vi "DRC Send Command.vi"(3 "error in (no error)":errorcluster, 4 "Input":dbl min=0.0 format="%.3f", 5 "StringInput":string, 6 "Command":T1(ring)) -> (0 "error out":errorcluster, 1 "Output":dbl format="%.2f", 2 "Response":string)   [LabVIEW 2019]
uses:
  GL_DRC_GPIBadd.vi
  GL_DRCtype.vi
  GL_DRCchannel.vi
panel:
  out "CHANNEL":bool
  out "CONTROLLER TYPE":bool
  out "GPIB Address":string
  # "setpoint, heater value"
  # "temperature,etc."
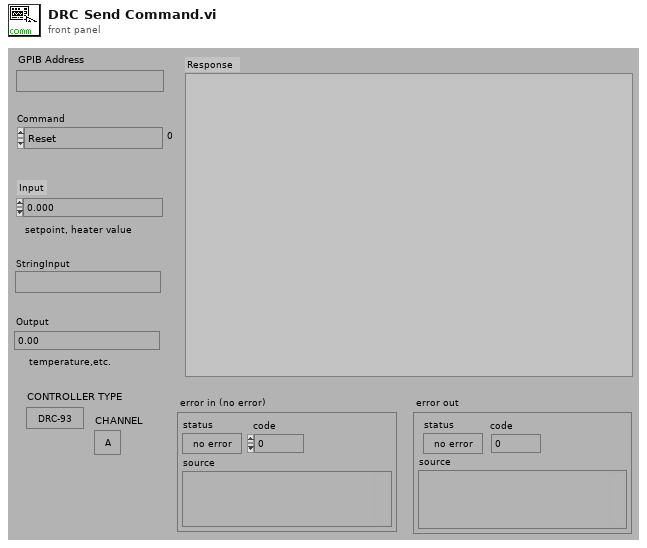
[diagram p1: front panel]
types:
  T1 = enum16{"Reset", "Raw_WriteRead", "ReadTemp", "WriteSetPoint", "ReadSetPoint", "ManualHeatPwr", "HeaterOff", "SetHeaterScale", "SetProportional(gain)", "SetIntegrate(reset)", "SetDerivative(rate)", "SendCalibration", "ReadCalibration", "SelectCurve", "GetControlInfo", "Change units", "GetDCSP_Reading", "GetPIDR_Reading", "ZeroNonVol_Mem"}
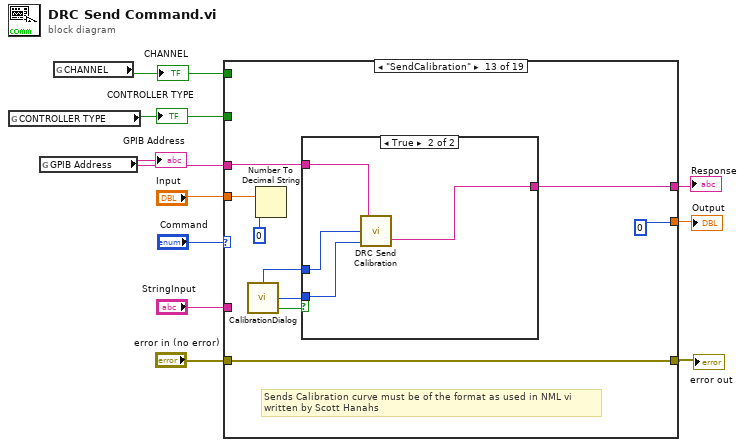
[diagram p0: block diagram]
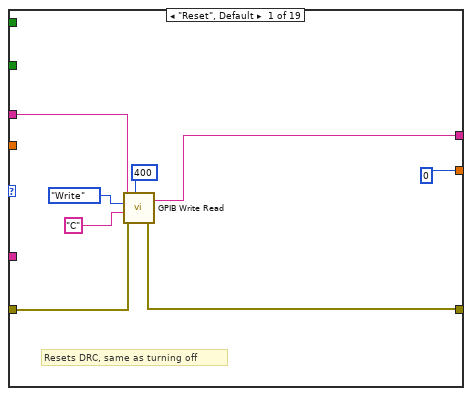
[diagram p2: hidden frame]
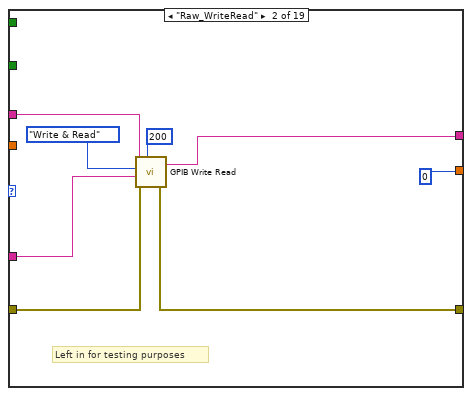
[diagram p3: hidden frame]
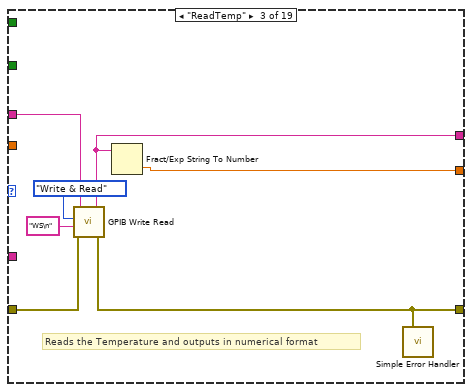
[diagram p4: hidden frame]
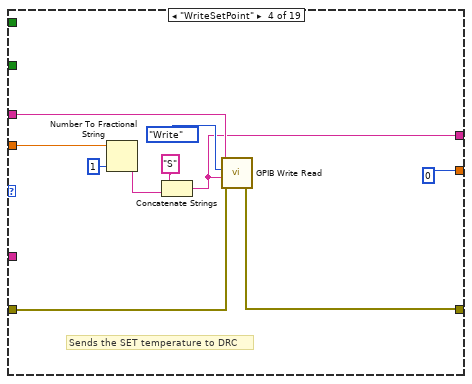
[diagram p5: hidden frame]
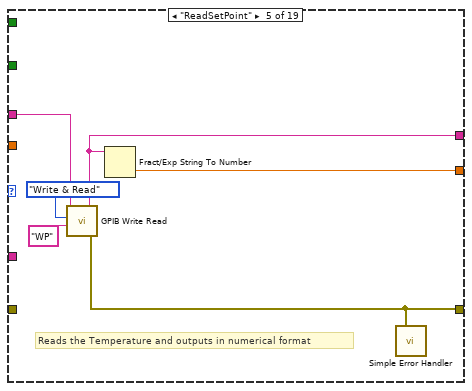
[diagram p6: hidden frame]
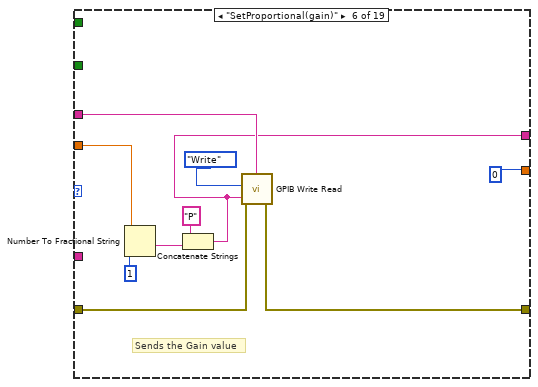
[diagram p7: hidden frame]
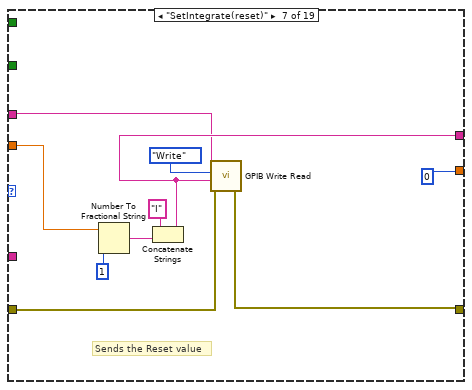
[diagram p8: hidden frame]
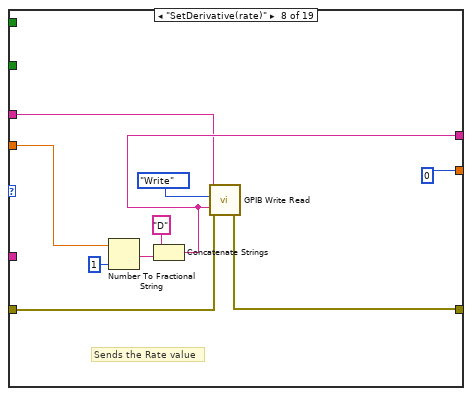
[diagram p9: hidden frame]
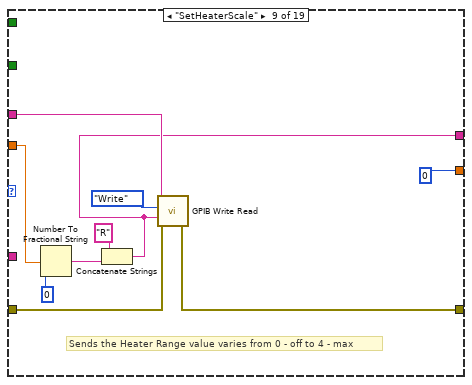
[diagram p10: hidden frame]
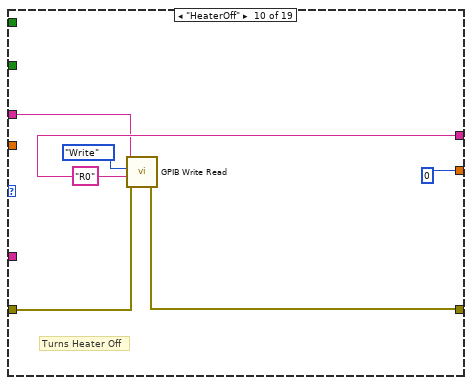
[diagram p11: hidden frame]
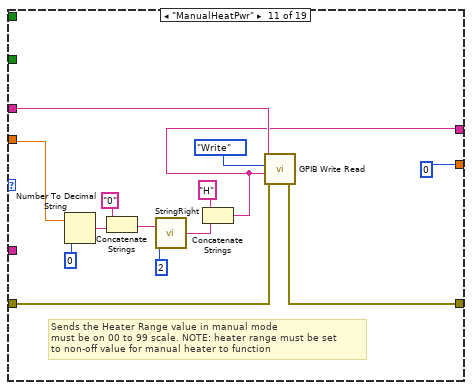
[diagram p12: hidden frame]
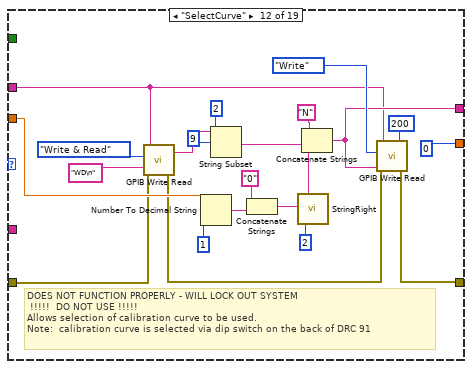
[diagram p13: hidden frame]
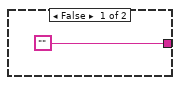
[diagram p14: hidden frame]
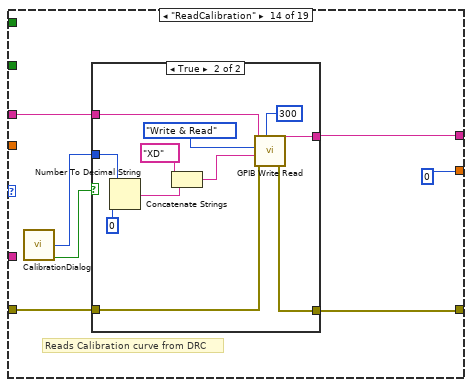
[diagram p15: hidden frame]
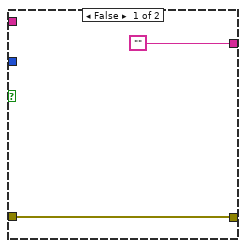
[diagram p16: hidden frame]
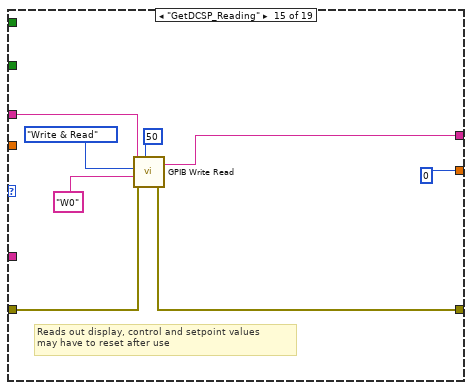
[diagram p17: hidden frame]
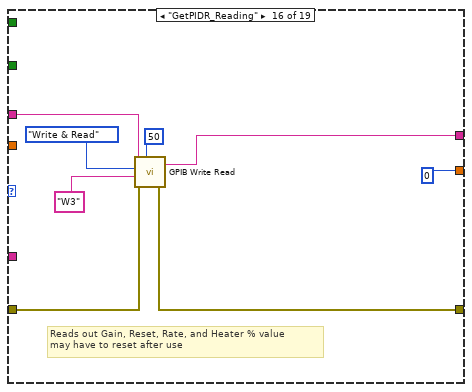
[diagram p18: hidden frame]
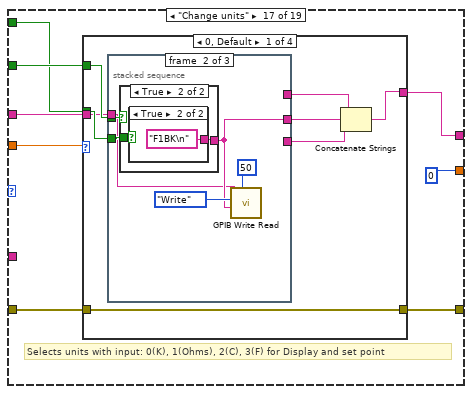
[diagram p19: hidden frame]
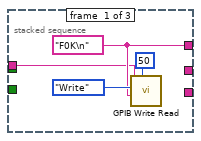
[diagram p20: hidden frame]
diagram:
  n1 = global read "GL_DRCtype.vi" "CONTROLLER TYPE"() -> (w2:bool)
  "CONTROLLER TYPE" <- w2
  n2 = global read "GL_DRC_GPIBadd.vi" "GPIB Address"() -> (w3:string)
  "GPIB Address" <- w3
  n3 = global read "GL_DRCchannel.vi" "CHANNEL"() -> (w1:bool)
  "CHANNEL" <- w1
  n4 = case shown="\"SendCalibration\"" "Command" {
    tunnel: [w15 w21 w30 w34 w46 w52 w64 w74 w82 w94 w98 w117 w137 w150 w168 w175 w184 w329 "Non-Volatile memory has been reinitialized"] -> w10
    tunnel: "StringInput" -> [_ w20 _ _ _ _ _ _ _ _ _ _ _ _ _ _ _ _ _]
    tunnel: "Input" -> [_ _ _ w38 _ w56 w66 w76 w86 _ w107 w122 w138 _ _ _ w189 _ _]
    tunnel: "error in (no error)" -> [w17 w23 w33 w37 _ w53 w62 w72 w83 w92 w99 w119 w136 w151 w170 w177 w188 w333 w340]
    tunnel: w2 -> [_ _ _ _ _ _ _ _ _ _ _ _ _ _ _ _ w187 w327 _]
    tunnel: w1 -> [_ _ _ _ _ _ _ _ _ _ _ _ _ _ _ _ w186 _ _]
    tunnel: [w12 w22 w27 w36 w44 w51 w61 w71 w81 w91 w97 w111 w136 w149 w169 w178 w185 w330 w338] -> w5
    tunnel: w3 -> [w18 w24 w31 w39 w49 w54 w63 w73 w84 w93 w100 w116 w140 w152 w171 w176 w183 w332 w341]
    tunnel: [0 0 w28 0 w45 0 0 0 0 0 0 0 0 0 0 0 0 0 0] -> w4
    frame "Reset", Default {
      # "Resets DRC, same as turning off"
      n5 = call "GPIB Write Read.vi"("GPIB address"=w18, "Action"=enum16{"Write", "Read", "Write & Read"}."Write" ("y"), "String to Write"="C" ("InputString"), "error in (no error)"=w17, "wait (mS)"=400) -> ("String Read"=w15:string, "error out"=w12:errorcluster)
    }
    frame "Raw_WriteRead" {
      # "Left in for testing purposes"
      n6 = call "GPIB Write Read.vi"("GPIB address"=w24, "Action"=enum16{"Write", "Read", "Write & Read"}."Write & Read", "String to Write"=w20, "error in (no error)"=w23, "wait (mS)"=200) -> ("String Read"=w21:string, "error out"=w22:errorcluster)
    }
    frame "ReadTemp" {
      # "Reads the Temperature and outputs in numerical format"
      n7 = call "GPIB Write Read.vi"("GPIB address"=w31, "Action"=enum16{"Write", "Read", "Write & Read"}."Write & Read", "String to Write"="WS\n", "error in (no error)"=w33) -> ("String Read"=w30:string, "error out"=w27:errorcluster)  [unwired: 1 in]
      n8 = Fract/Exp String To Number(string=w30) -> (number=w28:dbl)  [unwired: 3 in, 1 out]
      n9 = call <vilib>:"Simple Error Handler.vi"("error in (no error)"=w27) -> ()  [unwired: 4 in, 5 out]
    }
    frame "WriteSetPoint" {
      # "Sends the SET temperature to DRC"
      n10 = Number To Fractional String(number=w38, precision (6)=i16 1) -> (F-format string=w42:string)  [unwired: 2 in]
      n11 = Concatenate Strings("S", w42) -> (w34:string)
      n12 = call "GPIB Write Read.vi"("GPIB address"=w39, "Action"=enum16{"Write", "Read", "Write & Read"}."Write" ("y"), "String to Write"=w34, "error in (no error)"=w37) -> ("error out"=w36:errorcluster)  [unwired: 1 in, 1 out]
    }
    frame "ReadSetPoint" {
      # "Reads the Temperature and outputs in numerical format"
      n13 = call "GPIB Write Read.vi"("GPIB address"=w49, "Action"=enum16{"Write", "Read", "Write & Read"}."Write & Read", "String to Write"="WP") -> ("String Read"=w46:string, "error out"=w44:errorcluster)  [unwired: 2 in]
      n14 = Fract/Exp String To Number(string=w46) -> (number=w45:dbl)  [unwired: 3 in, 1 out]
      n15 = call <vilib>:"Simple Error Handler.vi"("error in (no error)"=w44) -> ()  [unwired: 4 in, 5 out]
    }
    frame "SetProportional(gain)" {
      # "Sends the Gain value"
      n16 = Number To Fractional String(number=w56, precision (6)=i16 1) -> (F-format string=w58:string)  [unwired: 2 in]
      n17 = Concatenate Strings("P", w58) -> (w52:string)
      n18 = call "GPIB Write Read.vi"("GPIB address"=w54, "Action"=enum16{"Write", "Read", "Write & Read"}."Write" ("y"), "String to Write"=w52, "error in (no error)"=w53) -> ("error out"=w51:errorcluster)  [unwired: 1 in, 1 out]
    }
    frame "SetIntegrate(reset)" {
      # "Sends the Reset value"
      n19 = Number To Fractional String(number=w66, precision (6)=i16 1) -> (F-format string=w68:string)  [unwired: 2 in]
      n20 = Concatenate Strings("I", w68) -> (w64:string)
      n21 = call "GPIB Write Read.vi"("GPIB address"=w63, "Action"=enum16{"Write", "Read", "Write & Read"}."Write" ("y"), "String to Write"=w64, "error in (no error)"=w62) -> ("error out"=w61:errorcluster)  [unwired: 1 in, 1 out]
    }
    frame "SetDerivative(rate)" {
      # "Sends the Rate value"
      n22 = Number To Fractional String(number=w76, precision (6)=i16 1) -> (F-format string=w78:string)  [unwired: 2 in]
      n23 = Concatenate Strings("D", w78) -> (w74:string)
      n24 = call "GPIB Write Read.vi"("GPIB address"=w73, "Action"=enum16{"Write", "Read", "Write & Read"}."Write" ("y"), "String to Write"=w74, "error in (no error)"=w72) -> ("error out"=w71:errorcluster)  [unwired: 1 in, 1 out]
    }
    frame "SetHeaterScale" {
      # "Sends the Heater Range value varies from 0 - off to 4 - max"
      n25 = Number To Fractional String(number=w86, precision (6)=i16 0) -> (F-format string=w88:string)  [unwired: 2 in]
      n26 = Concatenate Strings("R", w88) -> (w82:string)
      n27 = call "GPIB Write Read.vi"("GPIB address"=w84, "Action"=enum16{"Write", "Read", "Write & Read"}."Write" ("y"), "String to Write"=w82, "error in (no error)"=w83) -> ("error out"=w81:errorcluster)  [unwired: 1 in, 1 out]
    }
    frame "HeaterOff" {
      w94 = "R0"
      # "Turns Heater Off"
      n28 = call "GPIB Write Read.vi"("GPIB address"=w93, "Action"=enum16{"Write", "Read", "Write & Read"}."Write" ("y"), "String to Write"=w94, "error in (no error)"=w92) -> ("error out"=w91:errorcluster)  [unwired: 1 in, 1 out]
    }
    frame "ManualHeatPwr" {
      # "Sends the Heater Range value in manual mode \nmust be on 00 to 99 scale. NOTE: heater range must be set \nto non-off value for manual heater to function"
      n29 = Number To Decimal String(number=w107, width (-)=i16 0 ("precision (6)")) -> (decimal integer string=w103:string)
      n30 = Concatenate Strings("0" ("Substring"), w103) -> (w105:string)
      n31 = call "StringRight.vi"("#chars"=2, "input string"=w105) -> ("output string"=w102:string)  [unwired: 1 in]
      n32 = Concatenate Strings("H", w102) -> (w98:string)
      n33 = call "GPIB Write Read.vi"("GPIB address"=w100, "Action"=enum16{"Write", "Read", "Write & Read"}."Write" ("y"), "String to Write"=w98, "error in (no error)"=w99) -> ("error out"=w97:errorcluster)  [unwired: 1 in, 1 out]
    }
    frame "SelectCurve" {
      # "DOES NOT FUNCTION PROPERLY - WILL LOCK OUT SYSTEM\n !!!!!  DO NOT USE !!!!! \nAllows selection of calibration curve to be used.\nNote:  calibration curve is selected via dip switch on the back of DRC 91"
      n34 = call "GPIB Write Read.vi"("GPIB address"=w116, "Action"=enum16{"Write", "Read", "Write & Read"}."Write & Read", "String to Write"="WD\n", "error in (no error)"=w119) -> ("String Read"=w115:string, "error out"=w114:errorcluster)  [unwired: 1 in]
      n35 = Number To Decimal String(number=w122, width (-)=i16 1 ("precision (6)")) -> (decimal integer string=w121:string)
      n36 = String Subset(string=w115, offset (0)=9, length (rest)=2 ("length")) -> (substring=w126:string)
      n37 = Concatenate Strings("0" ("Substring"), w121) -> (w128:string)
      n38 = call "StringRight.vi"("#chars"=2, "input string"=w128) -> ("output string"=w125:string)  [unwired: 1 in]
      n39 = Concatenate Strings("N" ("Substring"), w126, w125) -> (w117:string)
      n40 = call "GPIB Write Read.vi"("GPIB address"=w116, "Action"=enum16{"Write", "Read", "Write & Read"}."Write" ("y"), "String to Write"=w117, "error in (no error)"=w114, "wait (mS)"=200 ("length")) -> ("error out"=w111:errorcluster)  [unwired: 1 out]
    }
    frame "SendCalibration" {
      # "Sends Calibration curve must be of the format as used in NML vi\nwritten by Scott Hanahs"
      n41 = call "CalibrationDialog.vi"() -> ("OK 2"=w133:bool, "Curve Number"=w132:i32, "Sensor Type display"=w134:i32)
      n42 = Number To Decimal String(number=w138, width (-)=i16 0 ("precision (6)")) -> ()  [unwired: 1 out]
      n43 = case shown="True" w133 {
        tunnel: w140 -> [_ w145]
        tunnel: ["" w144] -> w137
        tunnel: w134 -> [_ w143]
        tunnel: w132 -> [_ w142]
        frame False {
        }
        frame True {
          n44 = call "DRC Send Calibration.vi"("Calibration #"=w142, "Sensor Type"=w143, "GPIB Address (VISA)"=w145) -> ("Curve Table for this Calibration"=w144:string)  [unwired: 1 out]
        }
      }
    }
    frame "ReadCalibration" {
      # "Reads Calibration curve from DRC"
      n45 = call "CalibrationDialog.vi"() -> ("OK 2"=w146:bool, "Curve Number"=w147:i32)  [unwired: 1 out]
      n46 = case shown="True" w146 {
        tunnel: w152 -> [_ w161]
        tunnel: w147 -> [_ w159]
        tunnel: w151 -> [w154 w157]
        tunnel: [w154 w156] -> w149
        tunnel: ["" w155] -> w150
        frame False {
        }
        frame True {
          n47 = Number To Decimal String(number=w159, width (-)=i16 0 ("precision (6)")) -> (decimal integer string=w158:string)
          n48 = Concatenate Strings("XD", w158) -> (w164:string)
          n49 = call "GPIB Write Read.vi"("GPIB address"=w161, "Action"=enum16{"Write", "Read", "Write & Read"}."Write & Read", "String to Write"=w164, "error in (no error)"=w157, "wait (mS)"=i16 300 ("precision (6)")) -> ("String Read"=w155:string, "error out"=w156:errorcluster)
        }
      }
    }
    frame "GetDCSP_Reading" {
      # "Reads out display, control and setpoint values\nmay have to reset after use"
      n50 = call "GPIB Write Read.vi"("GPIB address"=w171, "Action"=enum16{"Write", "Read", "Write & Read"}."Write & Read", "String to Write"="W0", "error in (no error)"=w170, "wait (mS)"=50) -> ("String Read"=w168:string, "error out"=w169:errorcluster)
    }
    frame "GetPIDR_Reading" {
      # "Reads out Gain, Reset, Rate, and Heater % value\nmay have to reset after use"
      n51 = call "GPIB Write Read.vi"("GPIB address"=w176, "Action"=enum16{"Write", "Read", "Write & Read"}."Write & Read", "String to Write"="W3", "error in (no error)"=w177, "wait (mS)"=50) -> ("String Read"=w175:string, "error out"=w178:errorcluster)
    }
    frame "Change units" {
      # "Selects units with input: 0(K), 1(Ohms), 2(C), 3(F) for Display and set point"
      n52 = case shown="0, Default" w189 {
        tunnel: w188 -> [w195 w230 w262 w297]
        tunnel: w187 -> [w197 w229 w265 w295]
        tunnel: w186 -> [w196 w228 w261 w296]
        tunnel: [w195 w230 w262 w297] -> w185
        tunnel: [w193 w227 w263 w298] -> w184
        tunnel: w183 -> [w190 w224 w258 w292]
        frame 0, Default {
          n53 = stacked-sequence {
            tunnel: w197 -> [_ w205 w215]
            tunnel: w196 -> [_ w204 w214]
            tunnel: [w199 _ _] -> w194
            tunnel: [_ w203 _] -> w192
            tunnel: [_ _ w216] -> w191
            tunnel: w190 -> [w198 w202 w213]
            frame #0 {
              w199 = "F0K\n"
              n54 = call "GPIB Write Read.vi"("GPIB address"=w198, "Action"=enum16{"Write", "Read", "Write & Read"}."Write" ("y"), "String to Write"=w199, "wait (mS)"=50) -> ()  [unwired: 1 in, 2 out]
            }
            frame #1 {
              n55 = case shown="True" w205 {
                tunnel: ["F1K\n" w210] -> w203
                tunnel: w204 -> [_ w209]
                frame False {
                }
                frame True {
                  n56 = case shown="True" w209 {
                    tunnel: ["F1AK\n" "F1BK\n"] -> w210
                    frame False {
                    }
                    frame True {
                    }
                  }
                }
              }
              n57 = call "GPIB Write Read.vi"("GPIB address"=w202, "Action"=enum16{"Write", "Read", "Write & Read"}."Write" ("y"), "String to Write"=w203, "wait (mS)"=50) -> ()  [unwired: 1 in, 2 out]
            }
            frame #2 {
              n58 = case shown="True" w215 {
                tunnel: ["" w221] -> w216
                tunnel: w214 -> [_ w220]
                frame False {
                }
                frame True {
                  n59 = case shown="False" w220 {
                    tunnel: ["F2AK\n" "F2BK\n"] -> w221
                    frame False {
                    }
                    frame True {
                    }
                  }
                }
              }
              n60 = call "GPIB Write Read.vi"("GPIB address"=w213, "Action"=enum16{"Write", "Read", "Write & Read"}."Write" ("y"), "String to Write"=w216, "wait (mS)"=50) -> ()  [unwired: 1 in, 2 out]
            }
          }
          n61 = Concatenate Strings(w194, w192, w191) -> (w193:string)
        }
        frame 1 {
          n62 = stacked-sequence {
            tunnel: w229 -> [_ w239 w250]
            tunnel: w228 -> [_ w238 w249]
            tunnel: [w233 _ _] -> w231
            tunnel: [_ _ w248] -> w225
            tunnel: [_ w237 _] -> w226
            tunnel: w224 -> [w232 w236 w247]
            frame #0 {
              w233 = "F0S\n"
              n63 = call "GPIB Write Read.vi"("GPIB address"=w232, "Action"=enum16{"Write", "Read", "Write & Read"}."Write" ("y"), "String to Write"=w233, "wait (mS)"=50) -> ()  [unwired: 1 in, 2 out]
            }
            frame #1 {
              n64 = case shown="True" w239 {
                tunnel: ["F1S\n" w244] -> w237
                tunnel: w238 -> [_ w243]
                frame False {
                }
                frame True {
                  n65 = case shown="True" w243 {
                    tunnel: ["F1AS\n" "F1BS\n"] -> w244
                    frame False {
                    }
                    frame True {
                    }
                  }
                }
              }
              n66 = call "GPIB Write Read.vi"("GPIB address"=w236, "Action"=enum16{"Write", "Read", "Write & Read"}."Write" ("y"), "String to Write"=w237, "wait (mS)"=50) -> ()  [unwired: 1 in, 2 out]
            }
            frame #2 {
              n67 = case shown="True" w250 {
                tunnel: ["" w255] -> w248
                tunnel: w249 -> [_ w254]
                frame False {
                }
                frame True {
                  n68 = case shown="False" w254 {
                    tunnel: ["F2AS\n" "F2BS\n"] -> w255
                    frame False {
                    }
                    frame True {
                    }
                  }
                }
              }
              n69 = call "GPIB Write Read.vi"("GPIB address"=w247, "Action"=enum16{"Write", "Read", "Write & Read"}."Write" ("y"), "String to Write"=w248, "wait (mS)"=50) -> ()  [unwired: 1 in, 2 out]
            }
          }
          n70 = Concatenate Strings(w231, w226, w225) -> (w227:string)
        }
        frame 2 {
          n71 = stacked-sequence {
            tunnel: w265 -> [_ w273 w284]
            tunnel: w261 -> [_ w272 w283]
            tunnel: [w267 _ _] -> w264
            tunnel: [_ _ w282] -> w260
            tunnel: [_ w271 _] -> w259
            tunnel: w258 -> [w266 w270 w281]
            frame #0 {
              w267 = "F0C\n"
              n72 = call "GPIB Write Read.vi"("GPIB address"=w266, "Action"=enum16{"Write", "Read", "Write & Read"}."Write" ("y"), "String to Write"=w267, "wait (mS)"=50) -> ()  [unwired: 1 in, 2 out]
            }
            frame #1 {
              n73 = case shown="False" w273 {
                tunnel: ["F1C\n" w278] -> w271
                tunnel: w272 -> [_ w277]
                frame False {
                }
                frame True {
                  n74 = case shown="False" w277 {
                    tunnel: ["F1AC\n" "F1BC\n"] -> w278
                    frame False {
                    }
                    frame True {
                    }
                  }
                }
              }
              n75 = call "GPIB Write Read.vi"("GPIB address"=w270, "Action"=enum16{"Write", "Read", "Write & Read"}."Write" ("y"), "String to Write"=w271, "wait (mS)"=50) -> ()  [unwired: 1 in, 2 out]
            }
            frame #2 {
              n76 = case shown="True" w284 {
                tunnel: ["" w289] -> w282
                tunnel: w283 -> [_ w288]
                frame False {
                }
                frame True {
                  n77 = case shown="True" w288 {
                    tunnel: ["F2AC\n" "F2BC\n"] -> w289
                    frame False {
                    }
                    frame True {
                    }
                  }
                }
              }
              n78 = call "GPIB Write Read.vi"("GPIB address"=w281, "Action"=enum16{"Write", "Read", "Write & Read"}."Write" ("y"), "String to Write"=w282, "wait (mS)"=50) -> ()  [unwired: 1 in, 2 out]
            }
          }
          n79 = Concatenate Strings(w264, w259, w260) -> (w263:string)
        }
        frame 3 {
          n80 = stacked-sequence {
            tunnel: w295 -> [_ w307 w318]
            tunnel: w296 -> [_ w306 w317]
            tunnel: [w301 _ _] -> w299
            tunnel: [_ _ w316] -> w294
            tunnel: [_ w305 _] -> w293
            tunnel: w292 -> [w300 w304 w315]
            frame #0 {
              w301 = "F0F\n"
              n81 = call "GPIB Write Read.vi"("GPIB address"=w300, "Action"=enum16{"Write", "Read", "Write & Read"}."Write" ("y"), "String to Write"=w301, "wait (mS)"=50) -> ()  [unwired: 1 in, 2 out]
            }
            frame #1 {
              n82 = case shown="False" w307 {
                tunnel: ["F1F\n" w312] -> w305
                tunnel: w306 -> [_ w311]
                frame False {
                }
                frame True {
                  n83 = case shown="False" w311 {
                    tunnel: ["F1AF\n" "F1BF\n"] -> w312
                    frame False {
                    }
                    frame True {
                    }
                  }
                }
              }
              n84 = call "GPIB Write Read.vi"("GPIB address"=w304, "Action"=enum16{"Write", "Read", "Write & Read"}."Write" ("y"), "String to Write"=w305, "wait (mS)"=50) -> ()  [unwired: 1 in, 2 out]
            }
            frame #2 {
              n85 = case shown="True" w318 {
                tunnel: ["" w323] -> w316
                tunnel: w317 -> [_ w322]
                frame False {
                }
                frame True {
                  n86 = case shown="True" w322 {
                    tunnel: ["F2AF\n" "F2BF\n"] -> w323
                    frame False {
                    }
                    frame True {
                    }
                  }
                }
              }
              n87 = call "GPIB Write Read.vi"("GPIB address"=w315, "Action"=enum16{"Write", "Read", "Write & Read"}."Write" ("y"), "String to Write"=w316, "wait (mS)"=50) -> ()  [unwired: 1 in, 2 out]
            }
          }
          n88 = Concatenate Strings(w299, w293, w294) -> (w298:string)
        }
      }
    }
    frame "GetControlInfo" {
      # "Reads out sample, control and A and B input information\nmay have to reset after use"
      n89 = case shown="False" w327 {
        tunnel: ["WD\n" "W1\n"] -> w328
        frame False {
        }
        frame True {
        }
      }
      n90 = call "GPIB Write Read.vi"("GPIB address"=w332, "Action"=enum16{"Write", "Read", "Write & Read"}."Write & Read", "String to Write"=w328, "error in (no error)"=w333) -> ("String Read"=w329:string, "error out"=w330:errorcluster)  [unwired: 1 in]
    }
    frame "ZeroNonVol_Mem" {
      # "USE ONLY TO RESET NON-VOLATILE MEMORY\nALL DATA STORED CURVE # 08 TO 31"
      n91 = call "GPIB Write Read.vi"("GPIB address"=w341, "Action"=enum16{"Write", "Read", "Write & Read"}."Write", "String to Write"="XR&I*XR&I*XR&I*XR&I*XR&I*", "error in (no error)"=w340) -> ("error out"=w338:errorcluster)  [unwired: 1 in, 1 out]
    }
  }
  "Response" <- w10
  "error out" <- w5
  "Output" <- w4
